vi "Write DAC Voltage - All DUTs - All Channels.vi"(5 "Voltage":dbl format="%.3f V", 7 "Vref (-1: Unchanged)":dbl=-1.0 format="%.3f V", 11 "error in":errorcluster, 12 "Log (T)":bool=TRUE, 14 "FPGA":T1) -> (4 "Data Out":string[](array[string]), 15 "error out":errorcluster)   [LabVIEW 2017, in "Host SRL.lvlib"]
uses:
  Host SRL.lvlib
  Type Defs/WSVCAP SHL FPGA Enum.ctl
panel:
  # "With all 6 devices selected in the Device Map:\n\nThis VI will write to 1 Channel, 1 DUT on Each Device (6 DUTs Total)\n\nFor example, a DUT value of any of the following: 1,5,9,13,17,21\nAll of them will be written to"
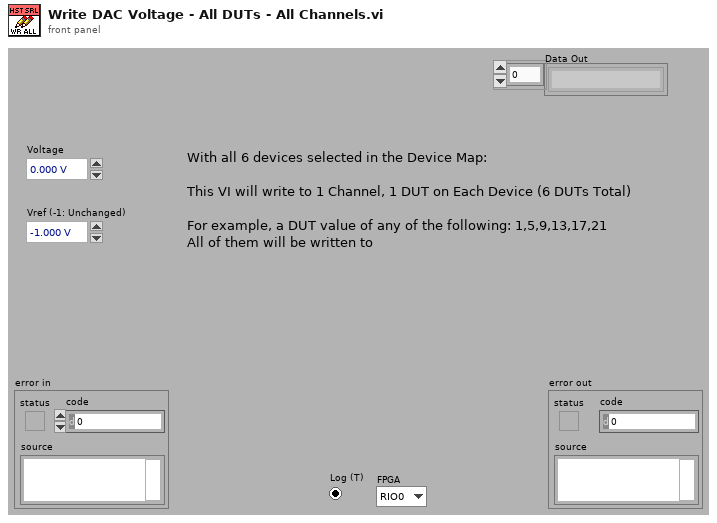
[diagram p1: front panel]
types:
  T1 = typedef "WSVCAP SHL FPGA Enum.ctl" = enum16{"RIO0", "RIO1"}
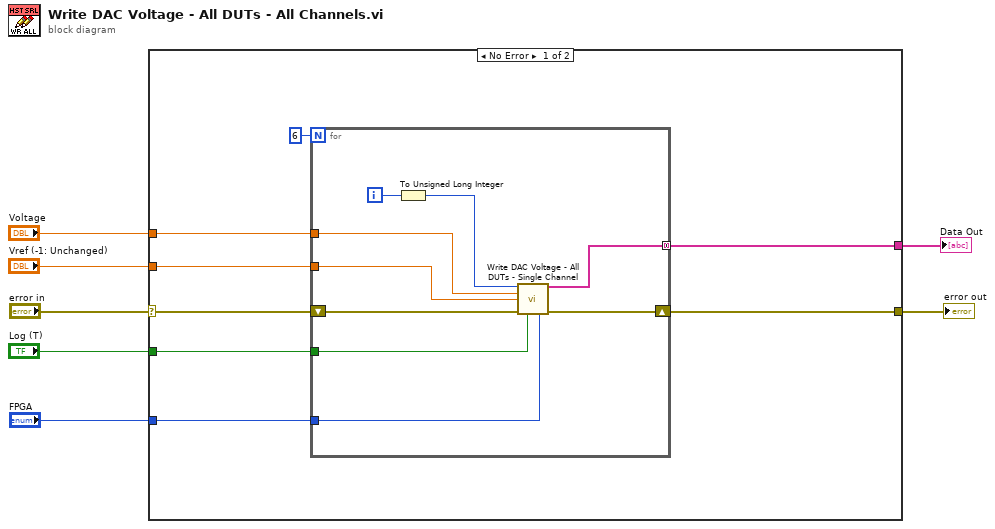
[diagram p0: block diagram]
diagram:
  n1 = case shown="No Error" "error in" {
    selector: "error in" -> [w12 _]
    tunnel: [w10 _] -> w7
    tunnel: "Log (T)" -> [w13 _]
    tunnel: "FPGA" -> [w14 _]
    tunnel: [w15 _] -> w3
    tunnel: "Voltage" -> [w9 _]
    tunnel: "Vref (-1: Unchanged)" -> [w11 _]
    frame No Error {
      n2 = for {
        N: 6 -> [_]
        tunnel: [w22] -> w15 mode=concatenating
        tunnel: w14 -> [w19]
        tunnel: w13 -> [w18]
        tunnel: w11 -> [w20]
        tunnel: w9 -> [w21]
        shift-right: [w23] -> w10
        shift-left: w12 -> [w24]
        i -> [w17]
        n3 = To Unsigned Long Integer(number=w17) -> (unsigned 32bit integer=w16:u32)
        n4 = call "Write DAC Voltage - All DUTs - Single Channel.vi"("Channel (0-5)"=w16, "Voltage"=w21, "Vref (-1: Unchanged)"=w20, "error in"=w24, "Log (T)"=w18, "FPGA"=w19) -> ("Data Out"=w22:string[], "error out"=w23:errorcluster)  [unwired: 8 in]
      }
    }
    frame Error {
    }
  }
  "error out" <- w7
  "Data Out" <- w3
